vi "VI Description Options.vi"(7 "Bookmark Options":T9={"Bookmarks as New Line in VI Descriptions"=TRUE, "Unique Bookmark Tags Only"=TRUE, "Include Tag and Text"=TRUE}, 8 "Error in":errorcluster caption="Error in (no error)", 11 "VI Info":T1) -> (0 "Error out":errorcluster, 3 "Description":string)   [LabVIEW 2023, in "VIDoc Printer.lvlib" / "VIDoc Printer.lvclass"]
doc: "Potentially appends Bookmark Tags to the description based on settings."
uses:
  VIDoc Printer.lvclass
  Settings/Printer Settings/Bookmark Options.ctl
  Parsing/TypeDefs/Method Spec Cluster.ctl
  Parsing/TypeDefs/VI Type Extended Enum.ctl
  <vilib>/picture/picture.llb/imagedata.ctl
  Parsing/TypeDefs/Class Dispatch Type Enum.ctl
  Parsing/TypeDefs/Controls Info Cluster.ctl
  <vilib>/Utility/miscctls.llb/LVKeyTypeDef.ctl
  <vilib>/Utility/miscctls.llb/LVPointTypeDef.ctl
  Parsing/SubVIs/Structure Reporter/Tree Cluster.ctl
  404875a6-21fa-4ea1-ab5b-c72591711ee0.vi
  <vilib>/Utility/error.llb/Trim Whitespace One-Sided.vi
  VIDoc Printer.lvclass/VIDoc Printer.ctl
  <userlib>/_PetranWay/LabVIEW Confluence API/Source/PetranWay_Confluence API.lvlib
  Settings/Printer Settings/Printer Settings.lvclass
  Parsing/VIDoc Parsing.lvlib
  Parsing/SubVIs/Structure Reporter/Structure Reporter.lvlib
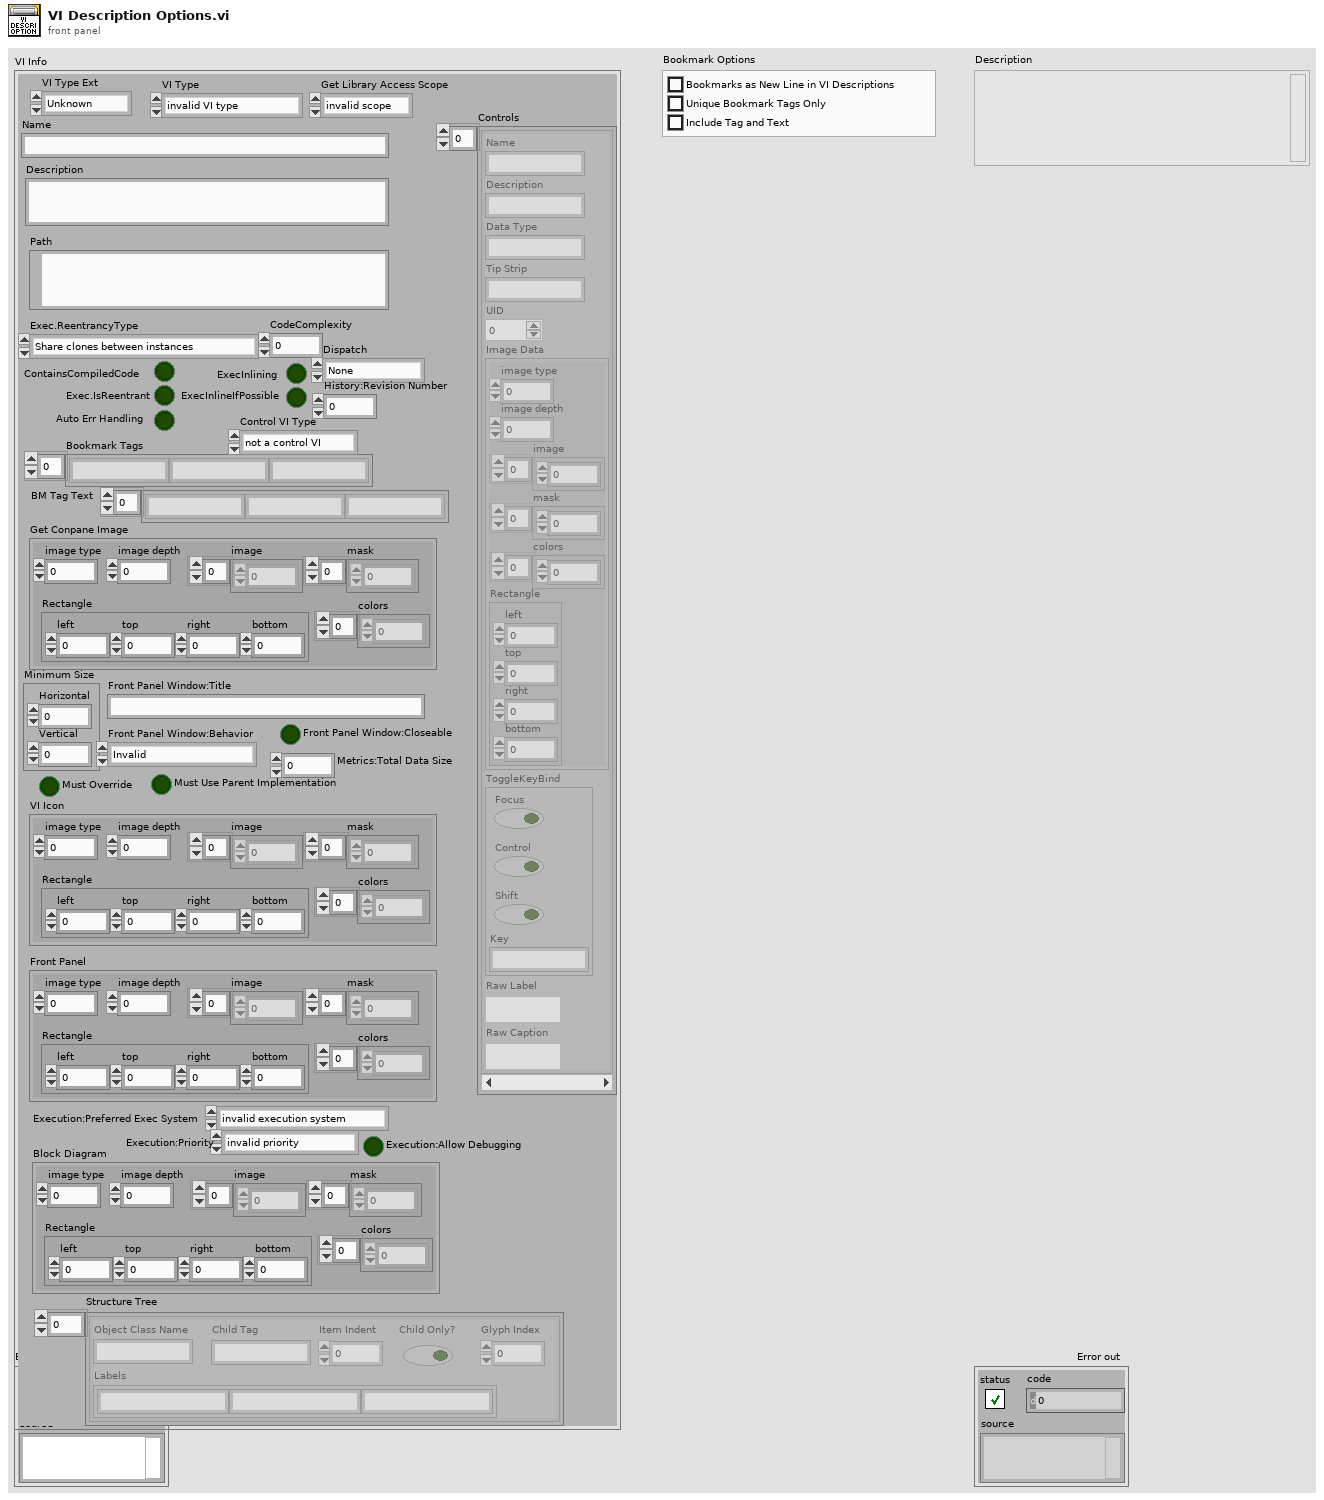
[diagram p1: front panel]
types:
  T1 = typedef "VIDoc Parsing.lvlib/Method Spec Cluster.ctl" = cluster{"VI Type Ext":T2, "Name":string, "Path":path, "Get Conpane Image":T3, "Description":string, "Get Library Access Scope":enum32{"invalid scope", "public", "private", "protected", "community"}, "Dispatch":T4, "ContainsCompiledCode":bool, "Exec.IsReentrant":bool, "Exec.ReentrancyType":enum16{"Share clones between instances", "Preallocate clone for each instance"}, "ExecInlining":bool, "ExecInlineIfPossible":bool, "Auto Err Handling":bool, "CodeComplexity":sgl, "Bookmark Tags":string[], "Control VI Type":enum32{"not a control VI", "control", "typedef", "strict typedef"}, "Controls":T5[], "VI Type":enum32{"invalid VI type", "Standard VI", "Control VI", "Global VI", "Polymorphic VI", "Configuration VI", "SubSystem", "Facade VI", "Method VI", "Statechart Diagram VI"}, "Minimum Size":T7, "Front Panel Window:Title":string, "Front Panel Window:Behavior":enum32{"Invalid", "Default", "Floating", "Floating/Auto-Hide", "Modal"}, "Front Panel Window:Closeable":bool, "Must Override":bool, "Must Use Parent Implementation":bool, "VI Icon":T3, "Front Panel":T3, "History:Revision Number":u32, "Metrics:Total Data Size":u32, "Execution:Allow Debugging":bool, "Execution:Preferred Exec System":enum32{"invalid execution system", "user interface", "standard", "instrument i/o", "data acquisition", "other 1", "other 2", "same as caller"}, "Execution:Priority":enum32{"invalid priority", "background priority", "normal priority", "above normal priority", "high priority", "time critical priority", "subroutine"}, "BM Tag Text":string[], "Block Diagram":T3, "Structure Tree":T8[]}
  T2 = typedef "VIDoc Parsing.lvlib/VI Type Extended Enum.ctl" = enum16{"Unknown", "Class Method", "Class Accessor Get", "Class Accessor Set", "Class Control", "Library Method", "Library Control", "VI", "Control"}
  T3 = typedef "imagedata.ctl" = cluster{"image type":i32, "image depth":i32, "image":u8[], "mask":u8[], "colors":u32[], "Rectangle":cluster{"left":i16, "top":i16, "right":i16, "bottom":i16}}
  T4 = typedef "VIDoc Parsing.lvlib/Class Dispatch Type Enum.ctl" = enum16{"None", "Static", "Dynamic"}
  T5 = typedef "VIDoc Parsing.lvlib/Controls Info Cluster.ctl" = cluster{"Name":string, "Description":string, "Data Type":string, "Tip Strip":string, "UID":i32, "Image Data":T3, "ToggleKeyBind":T6, "Raw Label":string, "Raw Caption":string}
  T6 = typedef "LVKeyTypeDef.ctl" = cluster{"Focus":bool, "Control":bool, "Shift":bool, "Key":string}
  T7 = typedef "LVPointTypeDef.ctl" = cluster{"Horizontal":i16, "Vertical":i16}
  T8 = typedef "VIDoc Parsing.lvlib/Structure Reporter.lvlib/Tree Cluster.ctl" = cluster{"Object Class Name":string, "Labels":string[], "Child Tag":string, "Item Indent":i32, "Child Only?":bool, "Glyph Index":i32}
  T9 = typedef "VIDoc Printer.lvlib/Printer Settings.lvclass/Bookmark Options.ctl" = cluster{"Bookmarks as New Line in VI Descriptions":bool, "Unique Bookmark Tags Only":bool, "Include Tag and Text":bool}
  T10 = cluster{"Bookmark Tag":string, "Bookmark Tag":string}
  T11 = cluster{"Bookmark Tag":string, "Bookmark Tag":string}[]
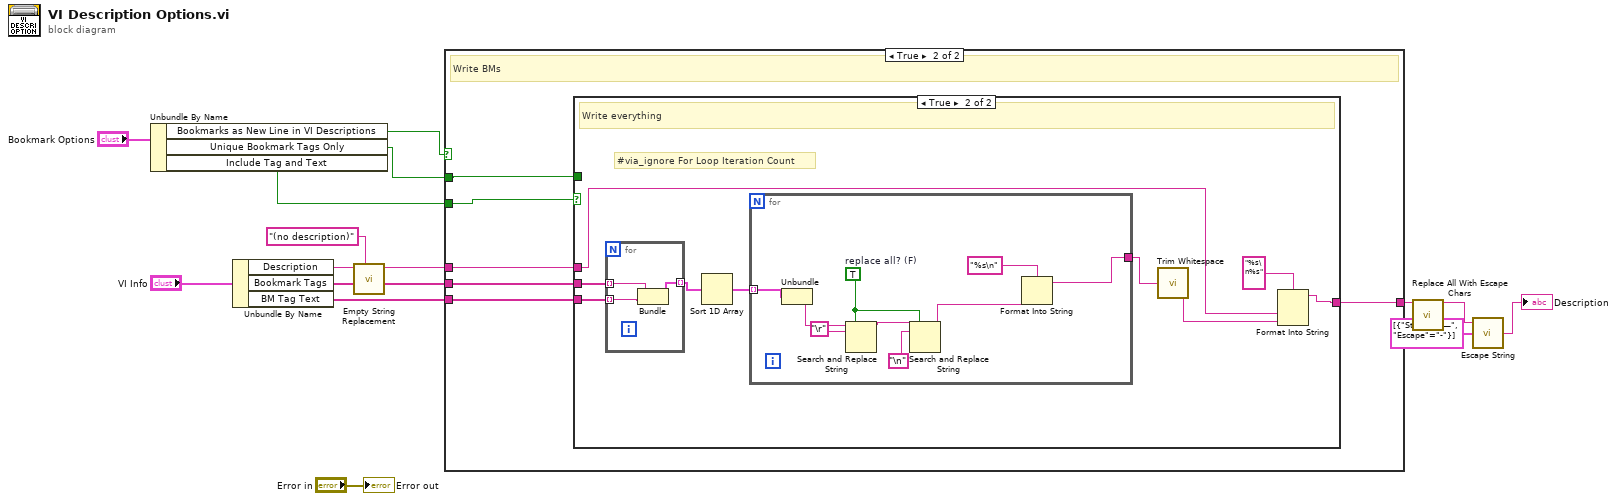
[diagram p0: block diagram]
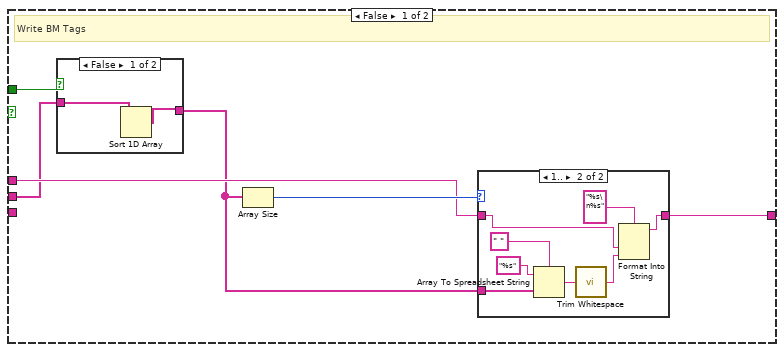
[diagram p3: hidden frame]
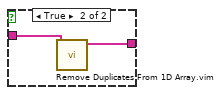
[diagram p4: hidden frame]
diagram:
  n1 = Unbundle By Name("Bookmark Options") -> ("Bookmarks as New Line in VI Descriptions"=w15:bool, "Unique Bookmark Tags Only"=w11:bool, "Include Tag and Text"=w10:bool)
  n2 = Unbundle By Name("VI Info") -> ("Description"=w13:string, "Bookmark Tags"=w12:string[], "BM Tag Text"=w9:string[])
  n3 = call "Empty String Replacement.vi"("Empty"="(no description)", "String"=w13) -> ("String Out"=w5:string)  [unwired: 9 in]
  n4 = case shown="True" w15 {
    tunnel: [w16 w22] -> w14
    tunnel: w5 -> [w16 w21]
    tunnel: w12 -> [_ w19]
    tunnel: w11 -> [_ w20]
    tunnel: w10 -> [_ w18]
    tunnel: w9 -> [_ w17]
    frame False {
    }
    frame True {
      # "Write BMs"
      n5 = case shown="True" w18 {
        tunnel: [w27 w45] -> w22
        tunnel: w21 -> [w26 w42]
        tunnel: w20 -> [w25 _]
        tunnel: w19 -> [w24 w50]
        tunnel: w17 -> [_ w49]
        frame False {
          # "Write BM Tags"
          n6 = case shown="False" w25 {
            tunnel: w24 -> [w30 w32]
            tunnel: [w29 w31] -> w23
            frame False {
              n7 = Sort 1D Array(array=w30) -> (sorted array=w29:string[])
            }
            frame True {
              n8 = call "Remove Duplicates From 1D Array.vim"("array"=w32) -> ("array with duplicates removed"=w31:string[])  [unwired: 10 in]
            }
          }
          n9 = Array Size(array=w23) -> (size(s)=w28:i32)
          n10 = case shown="1.." w28 {
            tunnel: [w33 w35] -> w27
            tunnel: w26 -> [w33 w37]
            tunnel: w23 -> [_ w41]
            frame 0, Default {
            }
            frame 1.. {
              n11 = Array To Spreadsheet String(delimiter (Tab)=" ", array=w41, 3:"%s" ("format string")) -> (spreadsheet string=w38:string)
              n12 = call <vilib>:"Trim Whitespace.vi"("string"=w38) -> ("trimmed string"=w36:string)  [unwired: 1 in]
              n13 = Format Into String(format string="%s\n%s", w37, w36) -> (resulting string=w35:string)  [unwired: 2 in, 1 out]
            }
          }
        }
        frame True {
          # "#via_ignore For Loop Iteration Count"
          # "Write everything"
          n14 = for {
            tunnel: w50 -> [w62] mode=indexing
            tunnel: w49 -> [w61] mode=indexing
            tunnel: [w60] -> w48 mode=indexing
            n15 = Bundle("Bookmark Tag"=w62, "Bookmark Tag"=w61) -> (w60:T10)  [unwired: 1 in]
          }
          n16 = Sort 1D Array(array=w48) -> (sorted array=w47:T11)
          n17 = for {
            tunnel: w47 -> [w59] mode=indexing
            tunnel: [w58] -> w44
            w54 = TRUE  # replace all? (F)
            n18 = Unbundle(w59) -> ("Bookmark Tag"=w57:string)  [unwired: 1 out]
            n19 = Search and Replace String(replace all?=w54, input string=w57, search string="\r") -> (result string=w56:string)  [unwired: 5 in, 3 out]
            n20 = Search and Replace String(replace all?=w54, input string=w56, search string="\n") -> (result string=w55:string)  [unwired: 5 in, 3 out]
            n21 = Format Into String(format string="%s\n", w55) -> (resulting string=w58:string)  [unwired: 2 in, 1 out]
          }
          n22 = call <vilib>:"Trim Whitespace.vi"("string"=w44) -> ("trimmed string"=w43:string)  [unwired: 1 in]
          n23 = Format Into String(format string="%s\n%s", w42, w43) -> (resulting string=w45:string)  [unwired: 2 in, 1 out]
        }
      }
    }
  }
  n24 = call <userlib>:"Replace All With Escape Chars.vi"("Raw String"=w14) -> ("With Substitued Escape Characters"=w3:string)  [unwired: 13 in, 1 out]
  n25 = call <vilib>:"Escape String.vi"("Escapes"=cluster{"String":string, "Escape":string}[] [{"String"="—", "Escape"="-"}], "String in"=w3) -> ("String out"=→"Description":string)  [unwired: 1 in]
  "Error out" <- "Error in"
